vi "Remove_Current_Active_Call.vi"(8 "error in (no error)":errorcluster, 10 "Elevator in":T1, 11 "Elevator Fleet in":T8) -> (0 "error out":errorcluster, 2 "Elevator out":T1, 3 "Elevator Fleet out":T8)   [LabVIEW 2026]
uses:
  Controls/Elevator_Status.ctl
  Controls/Door_Status_Enum.ctl
  Controls/Occupy_Status.ctl
  Controls/Floor_Status.ctl
  Controls/Motion_Status_Enum.ctl
  Controls/Car_Calls_Status.ctl
  Controls/Hall_Calls_Status.ctl
  Controls/Elevator_Fleet.ctl
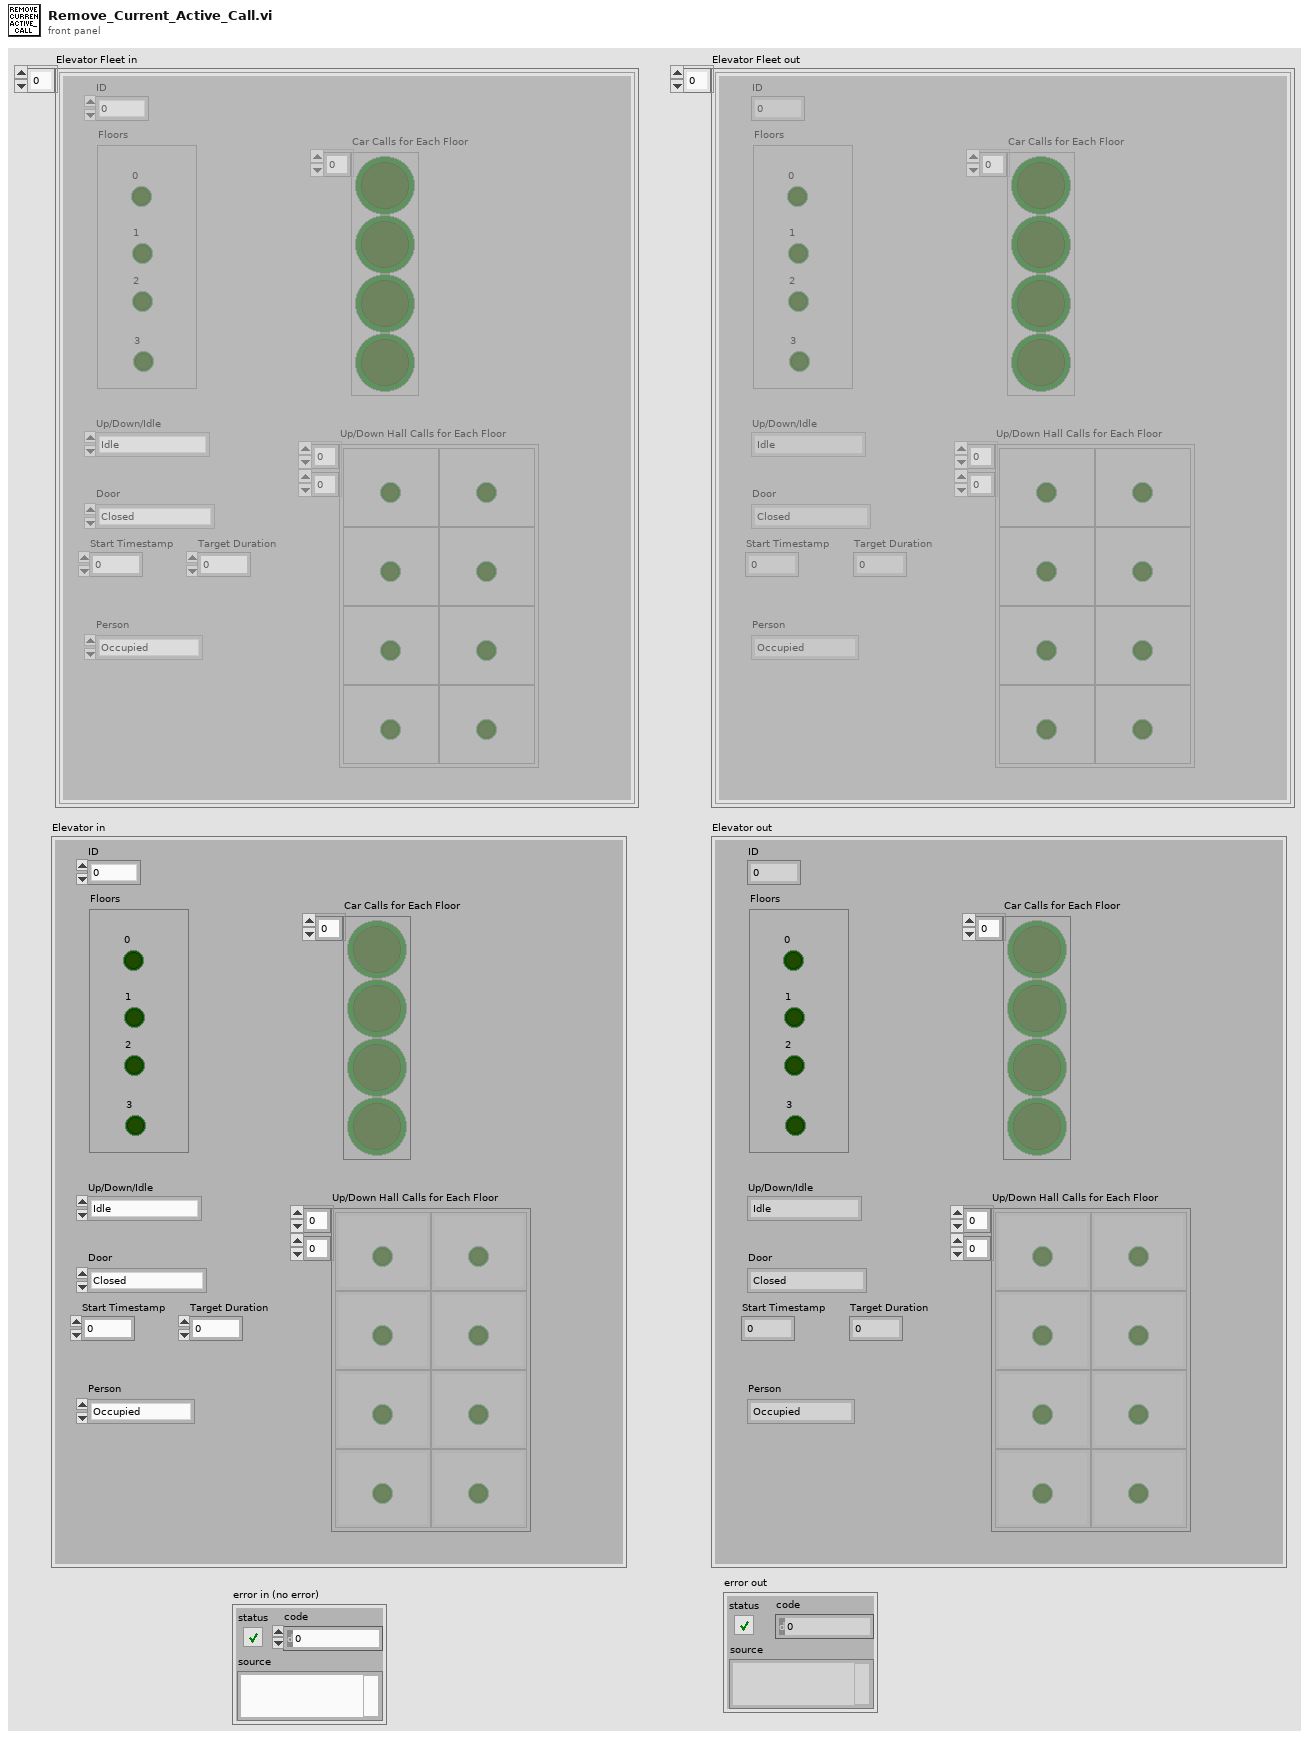
[diagram p1: front panel]
types:
  T1 = typedef "Elevator_Status.ctl" = cluster{"Door":T2, "Person":T3, "Floors":T4, "Up/Down/Idle":T5, "Car Calls for Each Floor":T6, "Up/Down Hall Calls for Each Floor":T7, "ID":i32, "Start Timestamp":u32, "Target Duration":dbl}
  T2 = typedef "Door_Status_Enum.ctl" = enum16{"Closed", "Open", "Opening", "Closing"}
  T3 = typedef "Occupy_Status.ctl" = enum16{"Occupied", "Empty"}
  T4 = typedef "Floor_Status.ctl" = cluster{"0":bool, "1":bool, "2":bool, "3":bool}
  T5 = typedef "Motion_Status_Enum.ctl" = enum16{"Idle", "Up", "Down"}
  T6 = typedef "Car_Calls_Status.ctl" = bool[]
  T7 = typedef "Hall_Calls_Status.ctl" = cluster{bool}[][]
  T8 = typedef "Elevator_Fleet.ctl" = T1[]
  T9 = enum16{"Check for Any Floor", "Check for Specific Floor"}
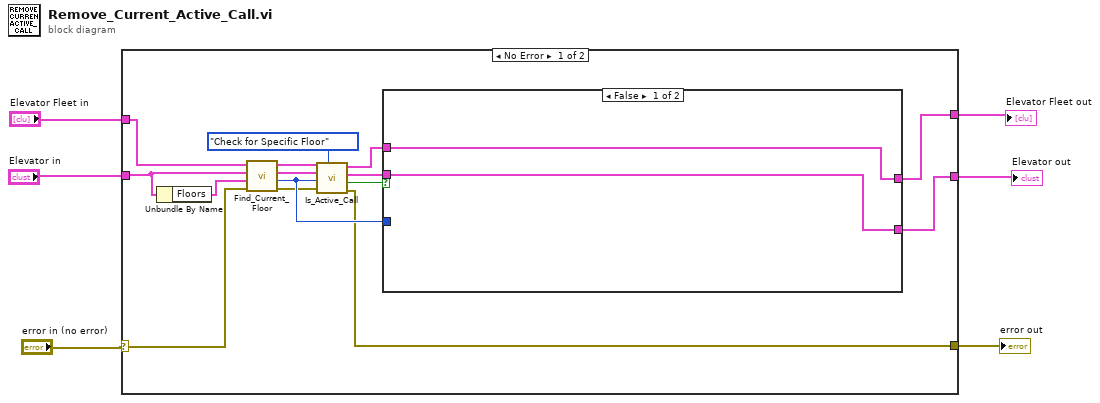
[diagram p0: block diagram]
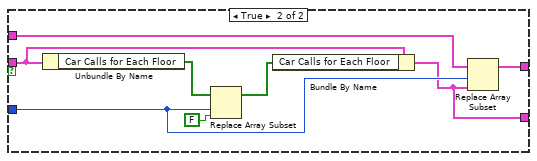
[diagram p2: hidden frame]
diagram:
  n1 = case shown="No Error" "error in (no error)" {
    selector: "error in (no error)" -> [w13 w34]
    tunnel: "Elevator in" -> [w10 w33]
    tunnel: "Elevator Fleet in" -> [w16 w32]
    tunnel: [w7 w33] -> w3
    tunnel: [w11 w34] -> w2
    tunnel: [w8 w32] -> w1
    frame No Error {
      n2 = Unbundle By Name(w10) -> ("Floors"=w14:T4)
      n3 = call "Find_Current_Floor.vi"("error in (no error)"=w13, "Floors"=w14, "Elevator Status in"=w10, "Elevator Fleet in"=w16) -> ("error out"=w12:errorcluster, "Current Floor"=w17:i32, "Elevator Status out"=w21:T1, "Elevator Fleet out"=w15:T8)  [unwired: 4 in]
      n4 = call "Is_Active_Call.vi"("Enum"=T9."Check for Specific Floor", "error in (no error)"=w12, "Floor"=w17, "Elevator in"=w21, "Elevator Fleet in"=w15) -> ("error out"=w11:errorcluster, "Active Call?"=w20:bool, "Elevator out"=w19:T1, "Elevator Fleet out"=w9:T8)  [unwired: 1 in]
      n5 = case shown="False" w20 {
        tunnel: w19 -> [w22 w29]
        tunnel: w17 -> [_ w27]
        tunnel: [w23 w25] -> w8
        tunnel: w9 -> [w23 w26]
        tunnel: [w22 w24] -> w7
        frame False {
        }
        frame True {
          n6 = Unbundle By Name(w29) -> ("Car Calls for Each Floor"=w31:T6)
          n7 = Replace Array Subset(array=w31, new element=FALSE ("new element/subarray"), index=w27) -> (w28:T6)
          n8 = Bundle By Name(cluster=w29, "Car Calls for Each Floor"=w28) -> (w24:T1)
          n9 = Replace Array Subset(array=w26, new element=w24, index=w27) -> (w25:T8)
        }
      }
    }
    frame Error {
    }
  }
  "Elevator Fleet out" <- w1
  "Elevator out" <- w3
  "error out" <- w2
